vi "RenderRobotSystemsDiagram.vi"(2 "Enable":bool, 3 "Cautions":bool[](array[boolean])=[FALSE, FALSE, FALSE, FALSE, FALSE, FALSE, FALSE, FALSE, FALSE, TRUE], 4 "Nominals":bool[](array[boolean])=[FALSE, FALSE, FALSE, FALSE, FALSE, FALSE, FALSE, FALSE, FALSE, TRUE], 5 "Alarms":bool[](array[boolean])=[FALSE, FALSE, FALSE, FALSE, FALSE, FALSE, FALSE, FALSE, FALSE, TRUE]) -> (1 "Robot Systems Diagram":T1(plugin-control))   [LabVIEW 2020]
uses:
  <vilib>/vision/NI_Vision_Development_Module.lvlib
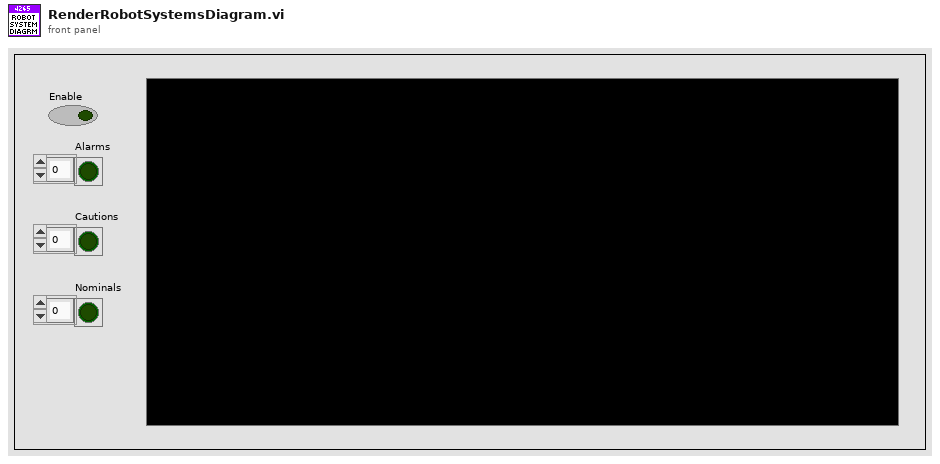
[diagram p1: front panel]
types:
  T1 = typedef "IMAQ Image.ctl" = refnum<image>
  T2 = typedef "imagedata.ctl" = cluster{"image type":i32, "image depth":i32, "image":u8[], "mask":u8[], "colors":u32[], "Rectangle":cluster{"left":i16, "top":i16, "right":i16, "bottom":i16}}
  T3 = typedef "Image Type" = u32
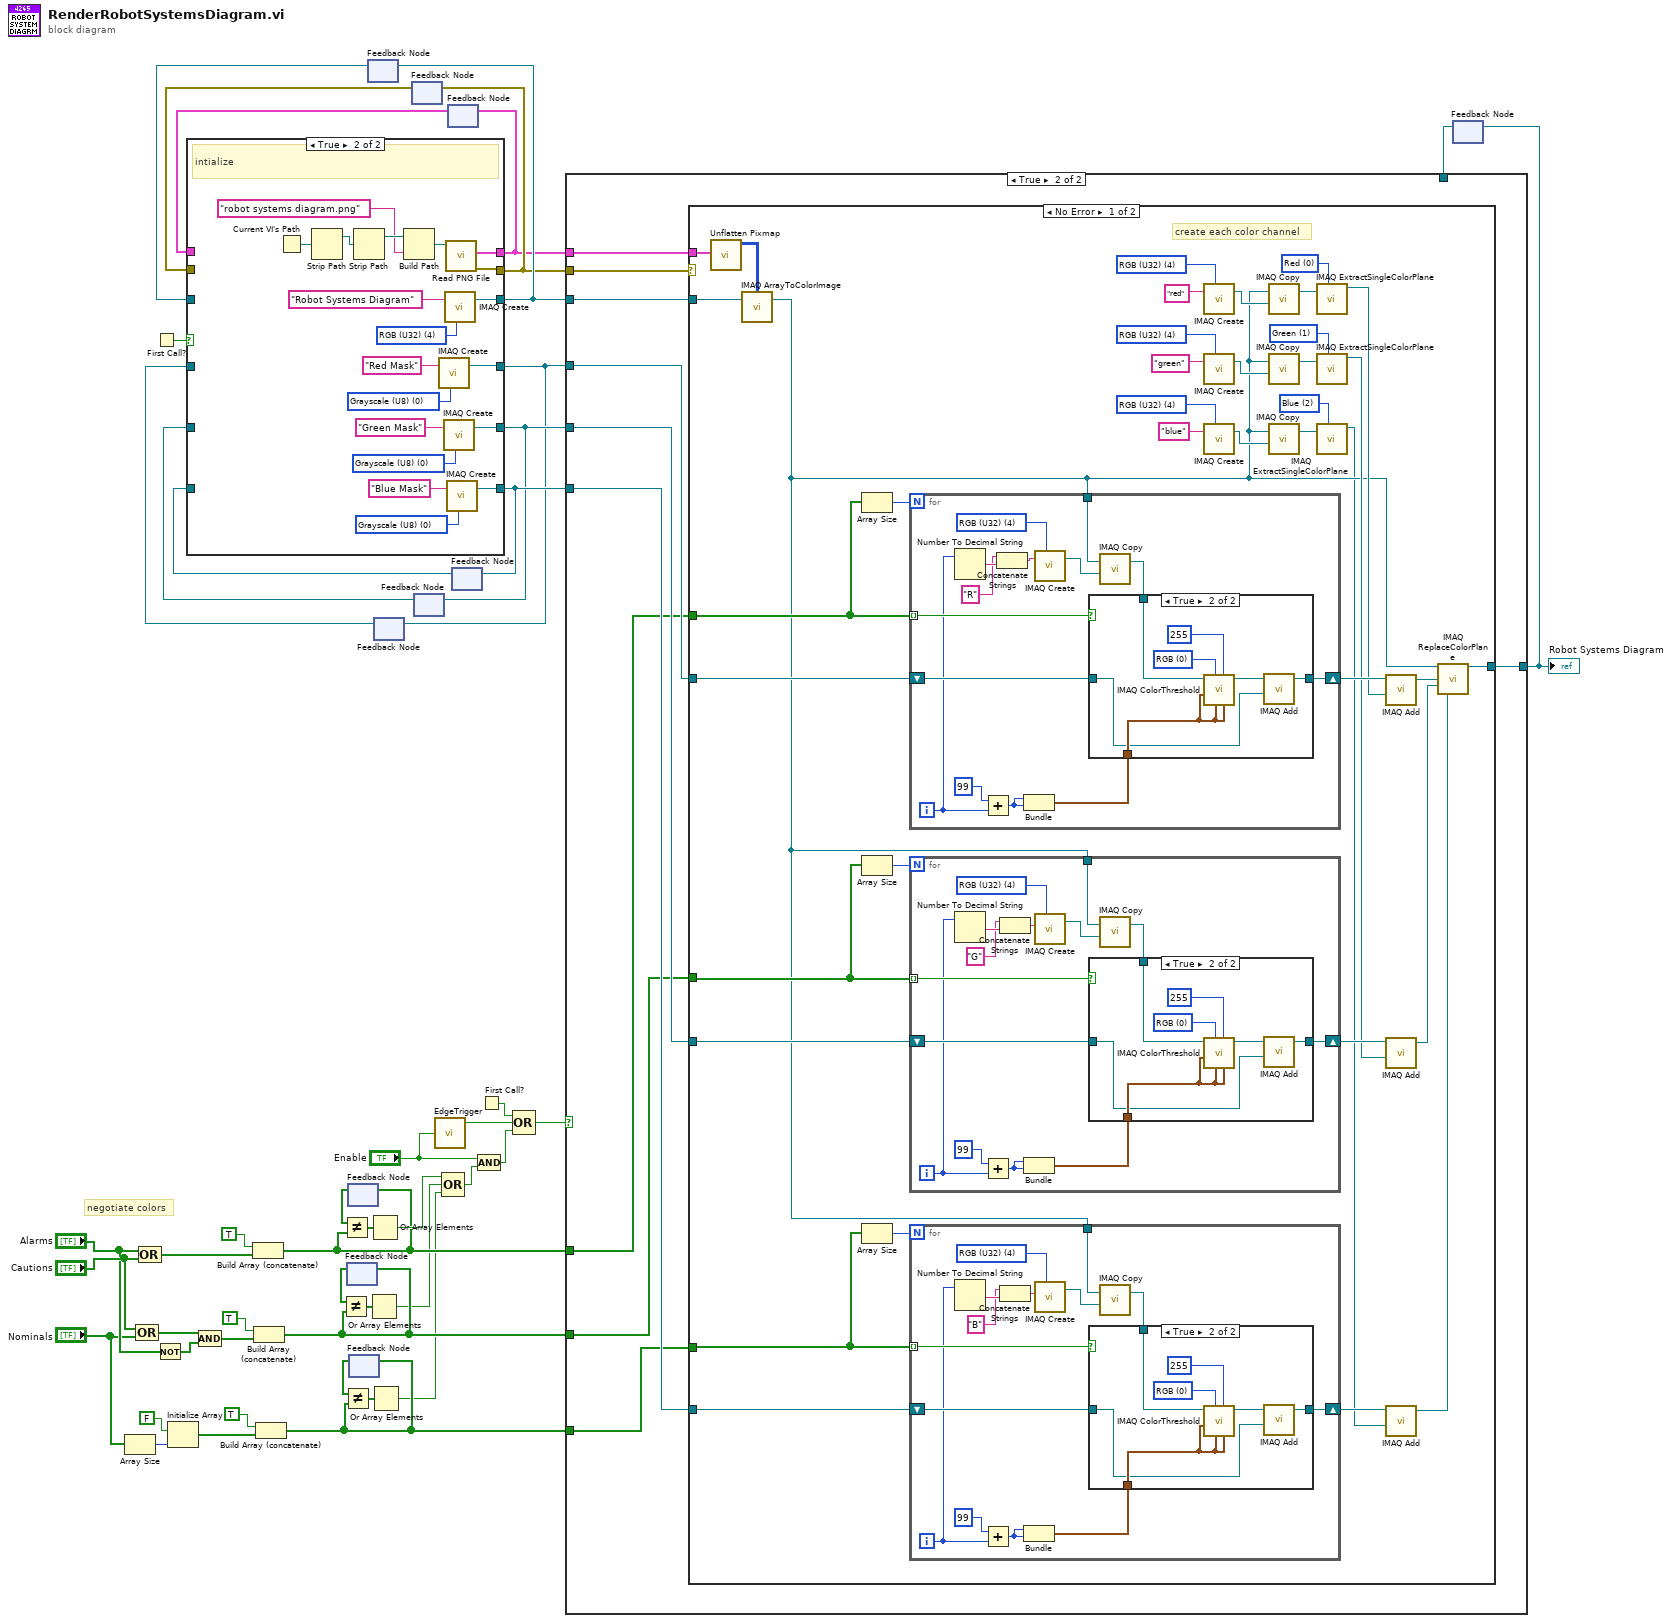
[diagram p0: block diagram]
diagram:
  # "negotiate colors"
  n1 = Array Size(array="Nominals") -> (size(s)=w29:i32)
  n2 = Compound Arithmetic op=OR("Cautions", "Nominals") -> (w33:bool[])
  n3 = Compound Arithmetic op=OR("Alarms", "Cautions") -> (w36:bool[])
  n4 = First Call?() -> (First Call?: T/F=w43:bool)
  n5 = Not(x="Alarms") -> (.not. x?=w32:bool[])
  n6 = Initialize Array(FALSE, w29) -> (w27:bool[])
  n7 = Compound Arithmetic op=AND(w33, w32) -> (w31:bool[])
  n8 = Build Array (concatenate)(TRUE, w36) -> (w17:bool[])
  n9 = Build Array (concatenate)(TRUE, w31) -> (w14:bool[])
  n10 = Build Array (concatenate)(TRUE, w27) -> (w11:bool[])
  n11 = feedback #1() -> (w16:bool[])  [unwired: 1 in]
  n12 = Not Equal?(x=w16, y=w14) -> (x != y?=w15:bool[])
  n13 = feedback-in #1(w14) -> ()
  n14 = feedback #2() -> (w20:bool[])  [unwired: 1 in]
  n15 = Not Equal?(x=w20, y=w17) -> (x != y?=w19:bool[])
  n16 = feedback-in #2(w17) -> ()
  n17 = feedback #3() -> (w13:bool[])  [unwired: 1 in]
  n18 = Not Equal?(x=w13, y=w11) -> (x != y?=w12:bool[])
  n19 = feedback-in #3(w11) -> ()
  n20 = feedback #4() -> (w41:T1)  [unwired: 1 in]
  n21 = Or Array Elements(Boolean array=w15) -> (logical OR=w10:bool)
  n22 = Or Array Elements(Boolean array=w19) -> (logical OR=w18:bool)
  n23 = Or Array Elements(Boolean array=w12) -> (logical OR=w9:bool)
  n24 = feedback #5() -> (w21:T1)  [unwired: 1 in]
  n25 = feedback #6() -> (w39:errorcluster)  [unwired: 1 in]
  n26 = feedback #7() -> (w23:T1)  [unwired: 1 in]
  n27 = call "EdgeTrigger.vi"("Input Signal"="Enable") -> ("Rising Edge Trigger"=w1:bool)  [unwired: 2 out]
  n28 = Compound Arithmetic op=OR(w18, w10, w9) -> (w8:bool)
  n29 = feedback #8() -> (w37:T2)  [unwired: 1 in]
  n30 = feedback #9() -> (w25:T1)  [unwired: 1 in]
  n31 = case shown="True" w43 {
    tunnel: [w52 w69] -> w42
    tunnel: w41 -> [w52 _]
    tunnel: [w51 w63] -> w40
    tunnel: [w50 w62] -> w38
    tunnel: w39 -> [w51 _]
    tunnel: w37 -> [w50 _]
    tunnel: [w47 w59] -> w22
    tunnel: [w48 w56] -> w24
    tunnel: [w49 w53] -> w26
    tunnel: w25 -> [w49 _]
    tunnel: w23 -> [w48 _]
    tunnel: w21 -> [w47 _]
    frame False {
    }
    frame True {
      w54 = T3 0 items=["Grayscale (U8)", "Grayscale (I16)", "Grayscale (SGL)", "Complex (CSG)", "RGB (U32)", "HSL (U32)", "RGB (U64)", "Grayscale (U16)"] ("Image Type")
      w57 = T3 0 items=["Grayscale (U8)", "Grayscale (I16)", "Grayscale (SGL)", "Complex (CSG)", "RGB (U32)", "HSL (U32)", "RGB (U64)", "Grayscale (U16)"] ("Image Type")
      w60 = T3 0 items=["Grayscale (U8)", "Grayscale (I16)", "Grayscale (SGL)", "Complex (CSG)", "RGB (U32)", "HSL (U32)", "RGB (U64)", "Grayscale (U16)"] ("Image Type")
      w70 = T3 4 items=["Grayscale (U8)", "Grayscale (I16)", "Grayscale (SGL)", "Complex (CSG)", "RGB (U32)", "HSL (U32)", "RGB (U64)", "Grayscale (U16)"] ("Image Type")
      # "intialize"
      n32 = Current VI's Path() -> (path=w65:path)
      n33 = Strip Path(path=w65) -> (stripped path=w66:path)  [unwired: 1 out]
      n34 = Strip Path(path=w66) -> (stripped path=w68:path)  [unwired: 1 out]
      n35 = Build Path(base path=w68, name or relative path="robot systems diagram.png") -> (appended path=w67:path)
      n36 = call "IMAQ Create"("Image Name"="Red Mask", "Image Type"=w60) -> ("New Image"=w59:T1)  [unwired: 3 in, 1 out]
      n37 = call "IMAQ Create"("Image Name"="Green Mask", "Image Type"=w57) -> ("New Image"=w56:T1)  [unwired: 3 in, 1 out]
      n38 = call "IMAQ Create"("Image Name"="Robot Systems Diagram", "Image Type"=w70) -> ("New Image"=w69:T1)  [unwired: 3 in, 1 out]
      n39 = call <vilib>:"Read PNG File.vi"("path to PNG file"=w67) -> ("error out"=w63:errorcluster, "image data"=w62:T2)  [unwired: 8 in, 1 out]
      n40 = call "IMAQ Create"("Image Name"="Blue Mask", "Image Type"=w54) -> ("New Image"=w53:T1)  [unwired: 3 in, 1 out]
    }
  }
  n41 = feedback-in #4(w42) -> ()
  n42 = feedback-in #5(w22) -> ()
  n43 = feedback-in #6(w40) -> ()
  n44 = feedback-in #7(w24) -> ()
  n45 = feedback-in #8(w38) -> ()
  n46 = feedback-in #9(w26) -> ()
  n47 = First Call?() -> (First Call?: T/F=w3:bool)
  n48 = Compound Arithmetic op=AND("Enable", w8) -> (w7:bool)
  n49 = Compound Arithmetic op=OR(w3, w1, w7) -> (w6:bool)
  n50 = feedback #10() -> (w4:T1)  [unwired: 1 in]
  n51 = case shown="True" w6 {
    tunnel: w42 -> [_ w82]
    tunnel: w40 -> [_ w81]
    tunnel: w38 -> [_ w80]
    tunnel: w26 -> [_ w79]
    tunnel: w24 -> [_ w78]
    tunnel: w22 -> [_ w77]
    tunnel: w17 -> [_ w76]
    tunnel: w14 -> [_ w75]
    tunnel: w11 -> [_ w74]
    tunnel: [w72 w73] -> w5
    tunnel: w4 -> [w72 _]
    frame False {
    }
    frame True {
      n52 = case shown="No Error" w81 {
        tunnel: w80 -> [w120 _]
        tunnel: [w97 w187] -> w73
        tunnel: w82 -> [w118 w187]
        tunnel: w76 -> [w117 _]
        tunnel: w77 -> [w116 _]
        tunnel: w75 -> [w93 _]
        tunnel: w78 -> [w92 _]
        tunnel: w74 -> [w84 _]
        tunnel: w79 -> [w83 _]
        frame No Error {
          w100 = 0 items=["Red", "Green", "Blue", "Hue", "Saturation", "Luminance", "Value", "Intensity"] ("Color Plane")
          w103 = T3 4 items=["Grayscale (U8)", "Grayscale (I16)", "Grayscale (SGL)", "Complex (CSG)", "RGB (U32)", "HSL (U32)", "RGB (U64)", "Grayscale (U16)"] ("Image Type")
          w105 = 1 items=["Red", "Green", "Blue", "Hue", "Saturation", "Luminance", "Value", "Intensity"] ("Color Plane")
          w108 = T3 4 items=["Grayscale (U8)", "Grayscale (I16)", "Grayscale (SGL)", "Complex (CSG)", "RGB (U32)", "HSL (U32)", "RGB (U64)", "Grayscale (U16)"] ("Image Type")
          w110 = 2 items=["Red", "Green", "Blue", "Hue", "Saturation", "Luminance", "Value", "Intensity"] ("Color Plane")
          w113 = T3 4 items=["Grayscale (U8)", "Grayscale (I16)", "Grayscale (SGL)", "Complex (CSG)", "RGB (U32)", "HSL (U32)", "RGB (U64)", "Grayscale (U16)"] ("Image Type")
          # "create each color channel"
          n53 = call <vilib>:"Unflatten Pixmap.vi"("image data"=w120) -> ("24-bit pixmap"=w119:u32[][])  [unwired: 4 in, 6 out]
          n54 = call "IMAQ ArrayToColorImage"("Image Pixels (U32)"=w119, "Image"=w118) -> ("Image Out"=w87:T1)  [unwired: 3 in, 1 out]
          n55 = Array Size(array=w117) -> (size(s)=w115:i32)
          n56 = Array Size(array=w93) -> (size(s)=w95:i32)
          n57 = Array Size(array=w84) -> (size(s)=w89:i32)
          n58 = for {
            N: w115 -> [_]
            tunnel: w117 -> [w176] mode=indexing
            shift-right: [w178] -> w114
            shift-left: w116 -> [w177]
            tunnel: w87 -> [w169]
            i -> [w171]
            w172 = T3 4 items=["Grayscale (U8)", "Grayscale (I16)", "Grayscale (SGL)", "Complex (CSG)", "RGB (U32)", "HSL (U32)", "RGB (U64)", "Grayscale (U16)"] ("Image Type")
            n59 = Number To Decimal String(number=w171) -> (decimal integer string=w166:string)  [unwired: 1 in]
            n60 = Add(x=99, y=w171) -> (x+y=w174:i32)
            n61 = Concatenate Strings("R" ("string"), w166) -> (w167:string)
            n62 = Bundle(w174, w174) -> (w173:cluster{i32, i32})  [unwired: 1 in]
            n63 = call "IMAQ Create"("Image Name"=w167, "Image Type"=w172) -> ("New Image"=w170:T1)  [unwired: 3 in, 1 out]
            n64 = call "IMAQ Copy"("Image Dst"=w170, "Image Src"=w169) -> ("Image Dst Out"=w168:T1)  [unwired: 4 in, 1 out]
            n65 = case shown="True" w176 {
              tunnel: [w179 w181] -> w178
              tunnel: w168 -> [_ w184]
              tunnel: w177 -> [w179 w180]
              tunnel: w173 -> [_ w183]
              frame False {
              }
              frame True {
                w186 = u16 0 items=["RGB", "HSL", "HSV", "HSI"] ("Color Mode")
                n66 = call "IMAQ ColorThreshold"("Blue or Luma or Val or Inten Range"=w183, "Replace Value"=255, "Green or Sat Range"=w183, "Color Mode"=w186, "Red or Hue Range"=w183, "Image Src"=w184) -> ("Image Dst Out"=w182:T1)  [unwired: 4 in, 1 out]
                n67 = call "IMAQ Add"("Image Src A"=w182, "Image Src B"=w180) -> ("Image Dst Out"=w181:T1)  [unwired: 5 in, 1 out]
              }
            }
          }
          n68 = for {
            N: w95 -> [_]
            tunnel: w93 -> [w154] mode=indexing
            shift-right: [w156] -> w94
            shift-left: w92 -> [w155]
            tunnel: w87 -> [w147]
            i -> [w149]
            w150 = T3 4 items=["Grayscale (U8)", "Grayscale (I16)", "Grayscale (SGL)", "Complex (CSG)", "RGB (U32)", "HSL (U32)", "RGB (U64)", "Grayscale (U16)"] ("Image Type")
            n69 = Number To Decimal String(number=w149) -> (decimal integer string=w145:string)  [unwired: 1 in]
            n70 = Add(x=99, y=w149) -> (x+y=w152:i32)
            n71 = Concatenate Strings("G" ("string"), w145) -> (w144:string)
            n72 = Bundle(w152, w152) -> (w151:cluster{i32, i32})  [unwired: 1 in]
            n73 = call "IMAQ Create"("Image Name"=w144, "Image Type"=w150) -> ("New Image"=w148:T1)  [unwired: 3 in, 1 out]
            n74 = call "IMAQ Copy"("Image Dst"=w148, "Image Src"=w147) -> ("Image Dst Out"=w146:T1)  [unwired: 4 in, 1 out]
            n75 = case shown="True" w154 {
              tunnel: [w157 w159] -> w156
              tunnel: w146 -> [_ w162]
              tunnel: w155 -> [w157 w158]
              tunnel: w151 -> [_ w161]
              frame False {
              }
              frame True {
                w164 = u16 0 items=["RGB", "HSL", "HSV", "HSI"] ("Color Mode")
                n76 = call "IMAQ ColorThreshold"("Blue or Luma or Val or Inten Range"=w161, "Replace Value"=255, "Green or Sat Range"=w161, "Color Mode"=w164, "Red or Hue Range"=w161, "Image Src"=w162) -> ("Image Dst Out"=w160:T1)  [unwired: 4 in, 1 out]
                n77 = call "IMAQ Add"("Image Src A"=w160, "Image Src B"=w158) -> ("Image Dst Out"=w159:T1)  [unwired: 5 in, 1 out]
              }
            }
          }
          n78 = for {
            N: w89 -> [_]
            tunnel: w84 -> [w132] mode=indexing
            shift-right: [w134] -> w88
            shift-left: w83 -> [w133]
            tunnel: w87 -> [w125]
            i -> [w127]
            w128 = T3 4 items=["Grayscale (U8)", "Grayscale (I16)", "Grayscale (SGL)", "Complex (CSG)", "RGB (U32)", "HSL (U32)", "RGB (U64)", "Grayscale (U16)"] ("Image Type")
            n79 = Number To Decimal String(number=w127) -> (decimal integer string=w123:string)  [unwired: 1 in]
            n80 = Add(x=99, y=w127) -> (x+y=w130:i32)
            n81 = Concatenate Strings("B" ("string"), w123) -> (w122:string)
            n82 = Bundle(w130, w130) -> (w129:cluster{i32, i32})  [unwired: 1 in]
            n83 = call "IMAQ Create"("Image Name"=w122, "Image Type"=w128) -> ("New Image"=w126:T1)  [unwired: 3 in, 1 out]
            n84 = call "IMAQ Copy"("Image Dst"=w126, "Image Src"=w125) -> ("Image Dst Out"=w124:T1)  [unwired: 4 in, 1 out]
            n85 = case shown="True" w132 {
              tunnel: [w135 w137] -> w134
              tunnel: w124 -> [_ w140]
              tunnel: w133 -> [w135 w136]
              tunnel: w129 -> [_ w139]
              frame False {
              }
              frame True {
                w142 = u16 0 items=["RGB", "HSL", "HSV", "HSI"] ("Color Mode")
                n86 = call "IMAQ ColorThreshold"("Blue or Luma or Val or Inten Range"=w139, "Replace Value"=255, "Green or Sat Range"=w139, "Color Mode"=w142, "Red or Hue Range"=w139, "Image Src"=w140) -> ("Image Dst Out"=w138:T1)  [unwired: 4 in, 1 out]
                n87 = call "IMAQ Add"("Image Src A"=w138, "Image Src B"=w136) -> ("Image Dst Out"=w137:T1)  [unwired: 5 in, 1 out]
              }
            }
          }
          n88 = call "IMAQ Create"("Image Name"="red", "Image Type"=w103) -> ("New Image"=w101:T1)  [unwired: 3 in, 1 out]
          n89 = call "IMAQ Create"("Image Name"="green", "Image Type"=w108) -> ("New Image"=w106:T1)  [unwired: 3 in, 1 out]
          n90 = call "IMAQ Create"("Image Name"="blue", "Image Type"=w113) -> ("New Image"=w111:T1)  [unwired: 3 in, 1 out]
          n91 = call "IMAQ Copy"("Image Dst"=w101, "Image Src"=w87) -> ("Image Dst Out"=w99:T1)  [unwired: 4 in, 1 out]
          n92 = call "IMAQ Copy"("Image Dst"=w106, "Image Src"=w87) -> ("Image Dst Out"=w104:T1)  [unwired: 4 in, 1 out]
          n93 = call "IMAQ Copy"("Image Dst"=w111, "Image Src"=w87) -> ("Image Dst Out"=w109:T1)  [unwired: 4 in, 1 out]
          n94 = call "IMAQ ExtractSingleColorPlane"("Color Plane"=w100, "Image Src"=w99) -> ("Image Dst Out"=w98:T1)  [unwired: 8 in, 1 out]
          n95 = call "IMAQ ExtractSingleColorPlane"("Color Plane"=w105, "Image Src"=w104) -> ("Image Dst Out"=w91:T1)  [unwired: 8 in, 1 out]
          n96 = call "IMAQ ExtractSingleColorPlane"("Color Plane"=w110, "Image Src"=w109) -> ("Image Dst Out"=w86:T1)  [unwired: 8 in, 1 out]
          n97 = call "IMAQ Add"("Image Src A"=w114, "Image Src B"=w98) -> ("Image Dst Out"=w96:T1)  [unwired: 5 in, 1 out]
          n98 = call "IMAQ Add"("Image Src A"=w94, "Image Src B"=w91) -> ("Image Dst Out"=w90:T1)  [unwired: 5 in, 1 out]
          n99 = call "IMAQ Add"("Image Src A"=w88, "Image Src B"=w86) -> ("Image Dst Out"=w85:T1)  [unwired: 5 in, 1 out]
          n100 = call "IMAQ ReplaceColorPlane"("Image Src"=w87, "Red or Hue Plane"=w96, "Green or Sat Plane"=w90, "Blue or Luma or Val or Inten Plane"=w85) -> ("Image Dst Out"=w97:T1)  [unwired: 10 in, 1 out]
        }
        frame Error {
        }
      }
    }
  }
  "Robot Systems Diagram" <- w5
  n101 = feedback-in #10(w5) -> ()
